vi "打开串口判定.vi"(8 "错误输入（无错误）":errorcluster, 11 "队列输入":refnum<queue>) -> ()   [LabVIEW 2016]
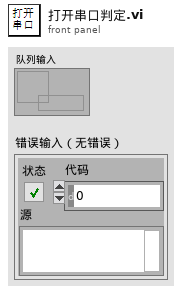
[diagram p1: front panel]
types:
  T1 = typedef "串口事件状态控件.ctl" = cluster{"串口状态":enum16{"打开串口", "关闭串口", "串口接收", "打开错误"}, "消息数据":variant}
  T2 = cluster{"串口状态":enum16{"打开串口", "关闭串口", "串口接收", "打开错误"}, "error IO":errorcluster}
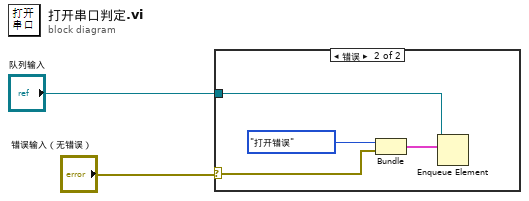
[diagram p0: block diagram]
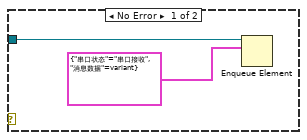
[diagram p2: hidden frame]
diagram:
  n1 = case shown="错误" "错误输入（无错误）" {
    selector: "错误输入（无错误）" -> [_ w8]
    tunnel: "队列输入" -> [w4 w7]
    frame No Error {
      n2 = Enqueue Element(queue=w4, element=T1 {"串口状态"=enum."串口接收", "消息数据"=variant}) -> ()  [unwired: 2 in, 3 out]
    }
    frame Error {
      n3 = Bundle("串口状态"=enum16{"打开串口", "关闭串口", "串口接收", "打开错误"}."打开错误", "error IO"=w8) -> (w5:T2)  [unwired: 1 in]
      n4 = Enqueue Element(queue=w7, element=w5) -> ()  [unwired: 2 in, 3 out]
    }
  }
